vi "Frequency Analysis of a Filter Design - DFD.vi"() -> ()   [LabVIEW 2023]
doc: "Demonstrates how to test the frequency response of a digital filter against arbitrary specifications. This example uses VIs in the LabVIEW Digital Filter Design Toolkit to design the filter and analyze the frequency response of the filter. The example then tests whether the result falls within the arbitrary limits. For this example, try changing the design parameters of the filter to successfully design a filter that passes the arbitrary specifications."
uses:
  <vilib>/measure/mamon.llb/Create Continuous Mask.vi
  <vilib>/addons/Digital Filter Design/Analysis.llb/DFD Plot Freq Response (Linear-Spaced).vi
  <vilib>/measure/mamon.llb/Limit Testing Frequency.vi
  <vilib>/measure/NI_MAPro.lvlib
  <vilib>/addons/Digital Filter Design/NI_DigFilterLicensed.lvlib
panel:
  in  "Filter specifications":T1={"Topology"=enum."Butterworth", "Type"=enum."Bandpass", "Order"=6, "Lower Fc"=2000.0, "Upper Fc"=3800.0, "PB Ripple"=0.025, "SB Attenuation"=90.0} {"PB Ripple" format="%0.4f"; "Lower Fc" format="%0.2p"; "SB Attenuation" format="%0.2f"; "Upper Fc" format="%0.2p"}
  in  "stop":bool
  out "Passed ?":bool
  out "Frequency Response":cluster{"x0":dbl, "dx":dbl, "Y":dbl[]}[](graph)
  # "Select Help»Show Context Help and move the cursor over the VI icon for more information."
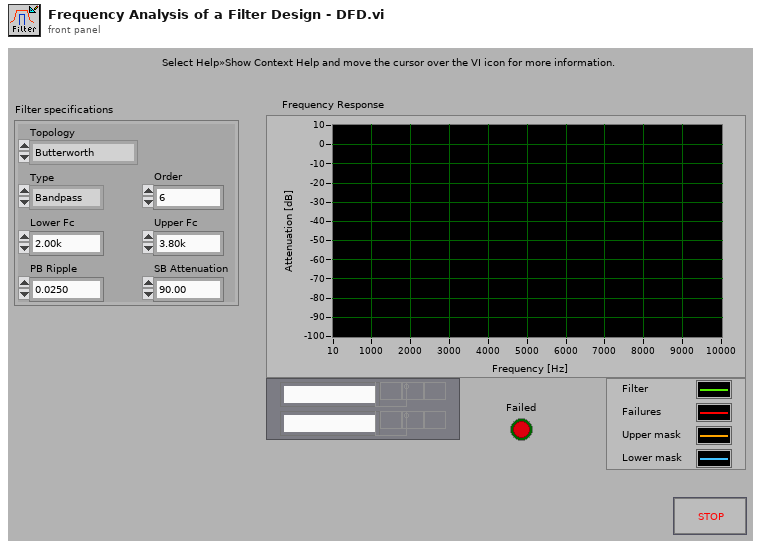
[diagram p1: front panel]
types:
  T1 = cluster{"Topology":enum16{"Off", "Butterworth", "Chebyshev", "Inverse Chebyshev", "Elliptic", "Bessel"}, "Type":enum16{"Lowpass", "Highpass", "Bandpass", "Bandstop"}, "Order":i32, "Lower Fc":dbl, "Upper Fc":dbl, "PB Ripple":dbl, "SB Attenuation":dbl}
  T2 = typedef "NI_DigFilterLicensed.lvlib/DFD Filter Obj.ctl" = cluster{"mSRate_Fs":dbl, "mSRate_Version":string, "mSRate_Comments":string, "mSRate_OrgCoef":T3, "mSRate_CurCoef":T3, "mSRate_Quantized?":bool, "mSRate_QCoef":T3, "mSRate_QSettings":T5[], "mSRate_Order":i32, "mSRate_Scaling":cluster{"mSRate_ScaleByPowerOf2?":bool, "mSRate_ScaleType":T7}}
  T3 = typedef "NI_DigFilterLicensed.lvlib/DFD Filter Coef.ctl" = cluster{"type":T4, "gain":dbl, "coef a (k)":dbl[], "coef b (v)":dbl[]}
  T4 = typedef "NI_DigFilterLicensed.lvlib/DFD Filter Structure Type Selector.ctl" = enum16{"Undefined", "FIR Direct Form", "FIR Direct Form Transposed", "FIR Symmetric", "FIR Antisymmetric", "IIR Direct Form I", "IIR Direct Form I Transposed", "IIR Direct Form II", "IIR Direct Form II Transposed", "IIR Cascaded Second Order Sections Form I", "IIR Cascaded Second Order Sections Form I Transposed", "IIR Cascaded Second Order Sections Form II", "IIR Cascaded Second Order Sections Form II Transposed", "Lattice Allpass (basic sections)", "Lattice Allpass (one multiplier sections)", "Lattice Allpass (normalized sections)", "Lattice AR (basic sections)", "Lattice AR (one multiplier sections)", "Lattice AR (normalized sections)", "Lattice MA (minimum phase)", "Lattice MA (maximum phase)", "Lattice ARMA (basic sections)", "Lattice ARMA (one multiplier sections)", "Lattice ARMA (normalized sections)"}
  T5 = typedef "NI_DigFilterLicensed.lvlib/dfd_Internal Quantization Settings.ctl" = cluster{"source":T6, "wl":i16, "iwl":i16, "overflow mode":enum16{"Saturation", "Wrap"}, "rounding mode":enum16{"Nearest", "Truncation"}, "signed?":bool}
  T6 = typedef "NI_DigFilterLicensed.lvlib/dfd_Internal Quantization Srcs.ctl" = u16
  T7 = typedef "NI_DigFilterLicensed.lvlib/DFD Coef Norm Type.ctl" = enum16{"No Norm", "Time Domain 1-Norm", "Time Domain 2-Norm", "Time Domain Inf-Norm"}
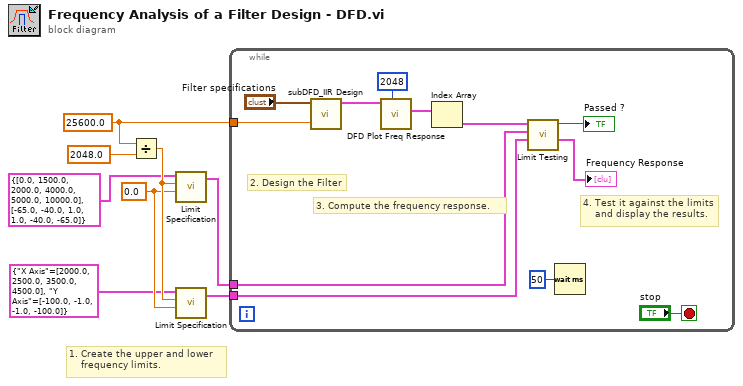
[diagram p0: block diagram]
diagram:
  w6 = 0.0 ("x0")
  w1 = 25600.0 ("Fs")
  # "1. Create the upper and lower \n    frequency limits."
  n1 = Divide(x=w1, y=2048.0 ("#s")) -> (x/y=w7:dbl)
  n2 = call-poly <vilib>:"Limit Specification.vi"("Specification Cluster"=cluster{dbl[], dbl[]} {[0.0, 1500.0, 2000.0, 4000.0, 5000.0, 10000.0], [-65.0, -40.0, 1.0, 1.0, -40.0, -65.0]} ("Output Cluster"), "dx"=w7, "x0"=w6) -> ("Limit"=w5:cluster{"x0":dbl, "dx":dbl, "Y":dbl[]})  [unwired: 2 in, 1 out]
  n3 = call-poly <vilib>:"Limit Specification.vi"("Specification Cluster"=cluster{"X Axis":dbl[], "Y Axis":dbl[]} {"X Axis"=[2000.0, 2500.0, 3500.0, 4500.0], "Y Axis"=[-100.0, -1.0, -1.0, -100.0]}, "dx"=w7, "x0"=w6) -> ("Limit"=w4:cluster{"x0":dbl, "dx":dbl, "Y":dbl[]})  [unwired: 2 in, 1 out]
  n4 = while {
    tunnel: w4 -> [w19]
    tunnel: w5 -> [w20]
    tunnel: w1 -> [w13]
    stop <- "stop" stop-if-true
    # "4. Test it against the limits\n    and display the results."
    # "3. Compute the frequency response."
    # "2. Design the Filter"
    n5 = call "subDFD_IIR Design.vi"("fs [Hz]"=w13, "Filter specifications"="Filter specifications") -> ("filter out"=w12:T2)  [unwired: 9 out]
    n6 = call-poly <vilib>:"DFD Plot Freq Response.vi"("# freq bins"=2048 ("# freq bins (auto)"), "filter in"=w12) -> ("magnitude response"=w10:cluster{"f0":dbl, "df":dbl, "values":dbl[]}[])  [unwired: 6 in, 3 out]
    n7 = Index Array(array=w10) -> (element=w9:cluster{"f0":dbl, "df":dbl, "values":dbl[]})  [unwired: 1 in]
    n8 = call-poly <vilib>:"Limit Testing.vi"("lower limit"=w19, "upper limit"=w20, "signal in"=w9) -> ("output values"=→"Frequency Response":cluster{"x0":dbl, "dx":dbl, "Y":dbl[]}[], "test passed?"=→"Passed ?":bool)  [unwired: 2 in, 5 out]
    n9 = Wait (ms)(milliseconds to wait=u32 50 ("millisecond multiple")) -> ()  [unwired: 1 out]
  }
